vi "Initialize.vi"(8 "error in (no error)":errorcluster, 11 "Channel in":refnum<class "Channel.lvclass">) -> (0 "error out":errorcluster, 3 "Channel out":refnum<class "Channel.lvclass">)   [LabVIEW 2018, in "Channel.lvclass"]
uses:
  Channel.lvclass
  Channel.lvclass/Channel.ctl
  Interface/Interface.lvclass
  StateMachine/State Machine.lvclass
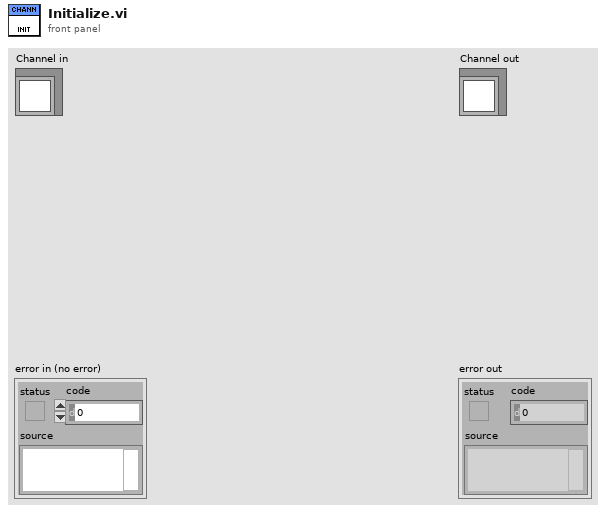
[diagram p1: front panel]
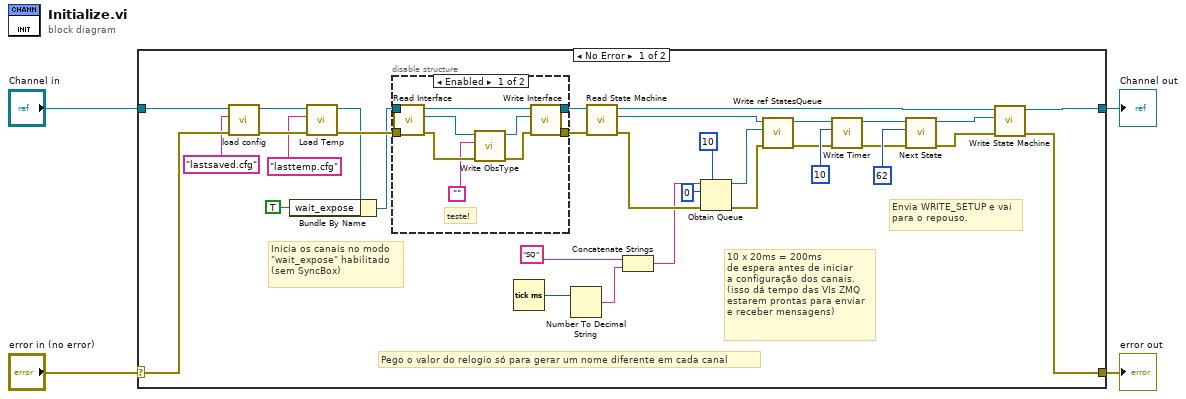
[diagram p0: block diagram]
diagram:
  n1 = case shown="No Error" "error in (no error)" {
    selector: "error in (no error)" -> [w30 w51]
    tunnel: [w33 w51] -> w3
    tunnel: [w34 w50] -> w1
    tunnel: "Channel in" -> [w31 w50]
    frame No Error {
      # "Pego o valor do relogio só para gerar um nome diferente em cada canal"
      # "Envia WRITE_SETUP e vai\npara o repouso."
      # "10 x 20ms = 200ms\nde espera antes de iniciar \na configuração dos canais.\n(isso dá tempo das VIs ZMQ\nestarem prontas para enviar\ne receber mensagens)"
      # "Inicia os canais no modo\n\"wait_expose\" habilitado\n(sem SyncBox)"
      n2 = call-dynamic "load config.vi"("error in (no error)"=w30, "cfg file name"="lastsaved.cfg", "Channel in"=w31) -> ("error out"=w25:errorcluster, "Channel out"=w26:refnum<class "Channel.lvclass">)  [unwired: 7 in]
      n3 = call-dynamic "Load Temp.vi"("error in (no error)"=w25, "temp file name"="lasttemp.cfg", "Channel in"=w26) -> ("error out"=w24:errorcluster, "Channel out"=w22:refnum<class "Channel.lvclass">)  [unwired: 7 in]
      n4 = Bundle By Name(cluster=w22, "wait_expose"=TRUE) -> (w21:refnum<class "Channel.lvclass">)
      n5 = disable-structure shown="Enabled" {
        disable-tunnel: w21 -> [w47 w49]
        disable-tunnel: [w45 w49] -> w28
        disable-tunnel: w24 -> [w42 w48]
        disable-tunnel: [w39 w48] -> w27
        frame Enabled {
          # "teste!"
          n6 = call-dynamic "Read Interface.vi"("error in (no error)"=w42, "Channel in"=w47) -> ("error out"=w41:errorcluster, "Interface.lvclass"=w44:refnum<class "Interface.lvclass">, "Channel out"=w46:refnum<class "Channel.lvclass">)  [unwired: 7 in]
          n7 = call-dynamic "Write ObsType.vi"("error in (no error)"=w41, "ObsType"="" ("Acq_Status"), "Interface in"=w44) -> ("error out"=w40:errorcluster, "Interface out"=w43:refnum<class "Interface.lvclass">)  [unwired: 7 in]
          n8 = call-dynamic "Write Interface.vi"("error in (no error)"=w40, "Interface.lvclass"=w43, "Channel in"=w46) -> ("error out"=w39:errorcluster, "Channel out"=w45:refnum<class "Channel.lvclass">)  [unwired: 7 in]
        }
        frame Disabled {
        }
      }
      n9 = Tick Count (ms)() -> (millisecond timer value=w8:u32)
      n10 = Number To Decimal String(number=w8) -> (decimal integer string=w6:string)  [unwired: 1 in]
      n11 = call-dynamic "Read State Machine.vi"("error in (no error)"=w27, "Device in"=w28) -> ("error out"=w15:errorcluster, "State Machine.lvclass"=w14:refnum<class "State Machine.lvclass">, "Device out"=w35:refnum<class "Channel.lvclass">)  [unwired: 7 in]
      n12 = Concatenate Strings("SQ" ("name (unnamed)"), w6) -> (w5:string)
      n13 = Obtain Queue(max queue size (-1, unlimited)=10, name (unnamed)=w5, element data type=u32 0 ("Timer"), error in (no error)=w15) -> (queue out=w12:refnum<queue>, error out=w11:errorcluster)  [unwired: 1 in, 1 out]
      n14 = call-dynamic "Write ref StatesQueue.vi"("error in (no error)"=w11, "ref StatesQueue"=w12, "State Machine in"=w14) -> ("error out"=w10:errorcluster, "State Machine out"=w13:refnum<class "State Machine.lvclass">)  [unwired: 7 in]
      n15 = call-dynamic "Write Timer.vi"("error in (no error)"=w10, "Timer"=u32 10, "State Machine in"=w13) -> ("error out"=w17:errorcluster, "State Machine out"=w18:refnum<class "State Machine.lvclass">)  [unwired: 7 in]
      n16 = call "Next State.vi"("error in (no error)"=w17, "New_State"=62, "State Machine in"=w18) -> ("error out"=w36:errorcluster, "State Machine out"=w37:refnum<class "State Machine.lvclass">)  [unwired: 7 in]
      n17 = call-dynamic "Write State Machine.vi"("error in (no error)"=w36, "State Machine.lvclass"=w37, "Device in"=w35) -> ("error out"=w33:errorcluster, "Device out"=w34:refnum<class "Channel.lvclass">)  [unwired: 7 in]
    }
    frame Error {
    }
  }
  "error out" <- w3
  "Channel out" <- w1
